vi "VariableGroupToggle.vi"(8 "error in (no error)":errorcluster, 9 "GroupName":string, 10 "VariableName":string, 11 "VMUI in":refnum<class "VMUI.lvclass">) -> (0 "error out":errorcluster, 3 "VMUI out":refnum<class "VMUI.lvclass">)   [LabVIEW 2013, in "VMUI.lvclass"]
doc: "Add a variable into a group, or remove a variable from a group if it already in the group.\nIf there is no group, nothing is done."
uses:
  VMUI.lvclass
  VariableManager/VariableManager.lvclass
  VariableGroup/VariableGroup.lvclass
  API/VariableManagerAPI.lvlib
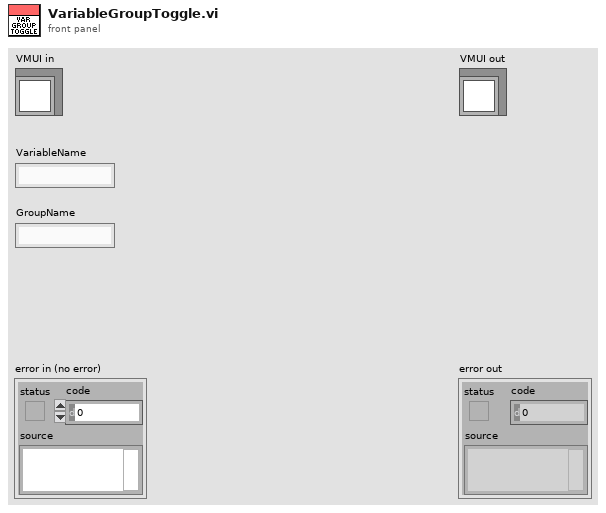
[diagram p1: front panel]
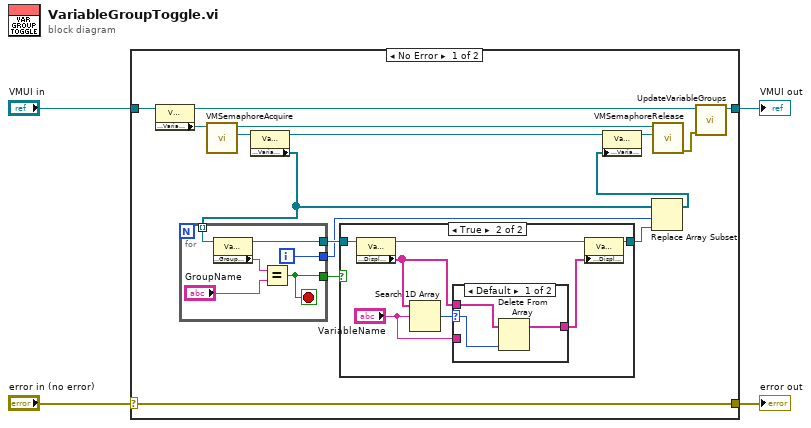
[diagram p0: block diagram]
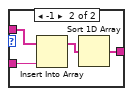
[diagram p3: hidden frame]
diagram:
  n1 = case shown="No Error" "error in (no error)" {
    selector: "error in (no error)" -> [w20 w43]
    tunnel: [w20 w43] -> w3
    tunnel: [w14 w42] -> w1
    tunnel: "VMUI in" -> [w19 w42]
    frame No Error {
      n2 = property class="VMUI.lvclass"(reference=w19) -> (reference out=w13:refnum<class "VMUI.lvclass">, "Accessors:VariableManagerRef"=w12:refnum<vi>)  [unwired: 1 in, 1 out]
      n3 = call "VMSemaphoreAcquire.vi"("VariableManagerRef in"=w12) -> ("VariableManager"=w7:refnum<class "VariableManager.lvclass">, "VariableManagerRef out"=w5:refnum<vi>)  [unwired: 7 in, 2 out]
      n4 = property class="VariableManager.lvclass"(reference=w7) -> (reference out=w10:refnum<class "VariableManager.lvclass">, "Accessors:VariableGroups"=w11:refnum<class "VariableGroup.lvclass">[])  [unwired: 1 in, 1 out]
      n5 = for {
        tunnel: w11 -> [w41] mode=indexing
        tunnel: [w38] -> w17
        tunnel: [w37] -> w16
        tunnel: [w36] -> w18
        i -> [w37]
        stop <- w36 stop-if-true
        n6 = property class="VariableGroup.lvclass"(reference=w41) -> (reference out=w38:refnum<class "VariableGroup.lvclass">, "Accessors:GroupName"=w40:string)  [unwired: 1 in, 1 out]
        n7 = Equal?(x=w40, y="GroupName") -> (x = y?=w36:bool)
      }
      n8 = case shown="True" w18 {
        tunnel: w17 -> [w21 w28]
        tunnel: [w21 w22] -> w15
        frame False {
        }
        frame True {
          n9 = property class="VariableGroup.lvclass"(reference=w28) -> (reference out=w24:refnum<class "VariableGroup.lvclass">, "Accessors:DisplayList"=w26:string[])  [unwired: 1 in, 1 out]
          n10 = Search 1D Array(1D array=w26, element="VariableName") -> (index of element=w27:i32)  [unwired: 1 in]
          n11 = case shown="Default" w27 {
            selector: w27 -> [w30 _]
            tunnel: w26 -> [w31 w35]
            tunnel: "VariableName" -> [_ w34]
            tunnel: [w29 w32] -> w23
            frame Default {
              n12 = Delete From Array(array=w31, index=w30) -> (array with subset deleted=w29:string[])  [unwired: 1 in, 1 out]
            }
            frame -1 {
              n13 = Insert Into Array(array=w35, new element=w34) -> (w33:string[])  [unwired: 1 in]
              n14 = Sort 1D Array(array=w33) -> (sorted array=w32:string[])
            }
          }
          n15 = property class="VariableGroup.lvclass"(reference=w24, "Accessors:DisplayList"=w23) -> (reference out=w22:refnum<class "VariableGroup.lvclass">)  [unwired: 1 in, 1 out]
        }
      }
      n16 = Replace Array Subset(array=w11, new element=w15, index=w16) -> (w9:refnum<class "VariableGroup.lvclass">[])
      n17 = property class="VariableManager.lvclass"(reference=w10, "Accessors:VariableGroups"=w9) -> (reference out=w6:refnum<class "VariableManager.lvclass">)  [unwired: 1 in, 1 out]
      n18 = call "VMSemaphoreRelease.vi"("VariableManager"=w6, "VariableManagerRef in"=w5) -> ("error out"=w8:errorcluster)  [unwired: 8 in, 1 out]
      n19 = call-dynamic "UpdateVariableGroups.vi"("error in (no error)"=w8, "VMUI in"=w13) -> ("VMUI out"=w14:refnum<class "VMUI.lvclass">)  [unwired: 8 in, 1 out]
    }
    frame Error {
    }
  }
  "error out" <- w3
  "VMUI out" <- w1
